vi "enqeue.vi"(10 "data":u64, 11 "on-board buffer in":T1) -> (3 "on-board buffer out":T1)   [LabVIEW 2010, in "OnBoardBuffer.lvlib"]
uses:
  OnBoardBuffer.lvlib
  OnBoardBuffer.ctl
  <vilib>/rvi/DataTransferAndStorage/Container/XNode/niFpgaContainer.xnode
  <vilib>/rvi/Memory/Memory_Emulation/nirvimemoryEmulationManagerCache_GetValue.vi
  <vilib>/rvi/DataTransferAndStorage/Container/Common/niFpgaContainerGetUniqueNameForEmu.vi
  <vilib>/rvi/Memory/Memory_Emulation/nirvimemoryEmulationManagerCache_InsertValue.vi
  <vilib>/Utility/error.llb/Clear Errors.vi
  <vilib>/rvi/Memory/Memory_Emulation/nirvimemoryEmulationManagerCache_SetValue.vi
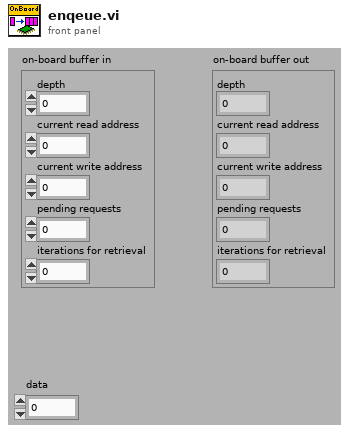
[diagram p1: front panel]
types:
  T1 = typedef "OnBoardBuffer.lvlib/OnBoardBuffer.ctl" = cluster{"depth":u32, "current read address":u32, "current write address":u32, "pending requests":u32, "iterations for retrieval":u32}
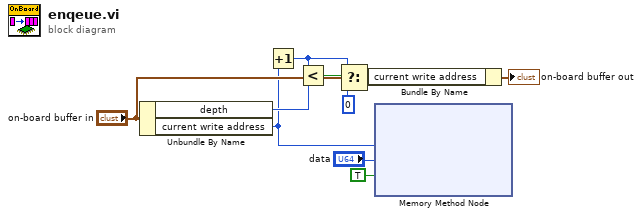
[diagram p0: block diagram]
diagram:
  n1 = Unbundle By Name("on-board buffer in") -> ("depth"=w10:u32, "current write address"=w3:u32)
  n2 = Increment(x=w3) -> (x+1=w7:u32)
  n3 = Less?(x=w7, y=w10) -> (x < y?=w9:bool)
  n4 = Select(t=w7, s=w9, f=u32 0) -> (s? t:f=w6:u32)
  n5 = Bundle By Name(cluster="on-board buffer in", "current write address"=w6) -> (→"on-board buffer out":T1)
  n6 = xnode ("Memory Method Node")("Address"=w3, "Data"="data", "Input Valid"=TRUE) -> ()  [unwired: 1 in, 2 out]
